vi "SS_Wait4Trigger.vi"(6 "Main Cluster IN":T1, 8 "Error In":errorcluster, 11 "Info In":string="\nWaiting for TimerScope Trigger\n- IN: SS TimerScope Trigger\n- OUT: SET SS ThermoRec Received Trigger\nPulse Number is 231123\nPulse Type is 4\n\nDuration (s) is  2.000000\nDelay (s)  is  1.000000\nScan Period (ms) is  15\nNumber of Samples is  134\n\nDelay Started\nDelay Complete\nExternal Measurement of Delay (s): 1.000000\nACQUIRING DATA") -> (0 "Error Out":errorcluster, 3 "Info Out":string="\nWaiting for TimerScope Trigger\n- IN: SS TimerScope Trigger\n- OUT: SET SS ThermoRec Received Trigger\nPulse Number is 231123\nPulse Type is 4\n\nDuration (s) is  2.000000\nDelay (s)  is  1.000000\nScan Period (ms) is  15\nNumber of Samples is  134\n\nDelay Started\nDelay Complete\nExternal Measurement of Delay (s): 1.000000\nACQUIRING DATA", 4 "Main Cluster OUT":T1)   [LabVIEW 2016]
uses:
  Control/Control_Main.ctl
  Control/Control_ModuleArray.ctl
  <vilib>/Platform/TimedLoop/XDataNode/timing_clust.ctl
  <vilib>/Platform/TimedLoop/XDataNode/nitl_modes.ctl
  <vilib>/Platform/TimedLoop/XDataNode/wakeup.ctl
  <vilib>/real-time/rtutility.llb/RT Restart Target (IP).vi
  <vilib>/Platform/TimedLoop/XDataNode/XDataNode.xnode
  <vilib>/Platform/TimedLoop/XDataNode/XDNodeRunTimeDep.lvlib
  <vilib>/real-time/NI_Real-Time Libraries.lvlib
panel:
  in  "Tab Control":enum32{"IN", "OUT", "SubVI Info"}(tab)
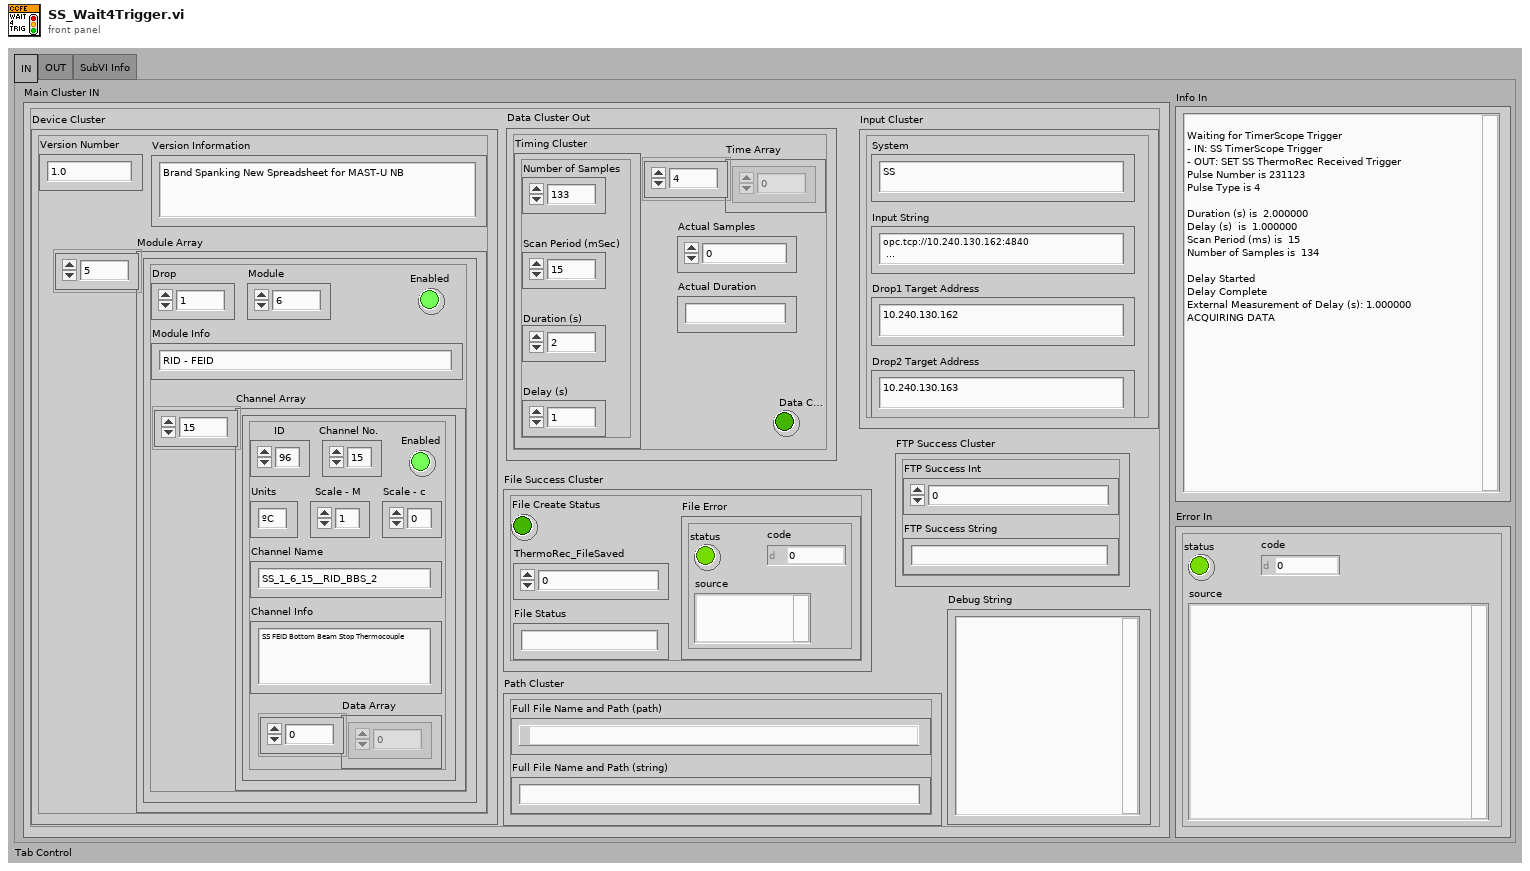
[diagram p1: front panel]
types:
  T1 = typedef "Control_Main.ctl" = cluster{"Device Cluster":cluster{"Module Array":T2, "Version Number":string, "Version Information":string}, "Input Cluster":cluster{"Input String":string, "Drop1 Target Address":string, "Drop2 Target Address":string, "System":string}, "Data Cluster Out":cluster{"Timing Cluster":cluster{"Number of Samples":i32, "Scan Period (mSec)":u32, "Duration (s)":dbl, "Delay (s)":dbl}, "Time Array":dbl[], "Actual Samples":i32, "Actual Duration":string, "Data Collection Error":bool}, "Path Cluster":cluster{"Full File Name and Path (path)":path, "Full File Name and Path (string)":string}, "File Success Cluster":cluster{"ThermoRec_FileSaved":i32, "File Create Status":bool, "File Error":errorcluster, "File Status":string}, "FTP Success Cluster":cluster{"FTP Success Int":i32, "FTP Success String":string}, "Debug String":string}
  T2 = typedef "Control_ModuleArray.ctl" = cluster{"Drop":i32, "Module":i32, "Module Info":string, "Enabled":bool, "Channel Array":cluster{"ID":i32, "Channel No.":i32, "Enabled":bool, "Channel Name":string, "Channel Info":string, "Units":string, "Scale - M":dbl, "Scale - c":dbl, "Data Array":dbl[]}[]}[]
  T3 = typedef "XDNodeRunTimeDep.lvlib/timing_clust.ctl" = cluster{"Expected End [f-1]":u64, "Actual End [f-1]":u64, "Finished Late? [f-1]":bool, "Expected End [i-1]":u64, "Actual End [i-1]":u64, "Finished Late? [i-1]":bool, "Expected Start [i]":u64, "Actual Start [i]":u64, "Expected Start [f]":u64, "Actual Start [f]":u64, "Source Name":string, "Structure Name":string, "Period":i64, "Deadline":i64, "Offset":i64, "Start":i64, "Priority":i32, "Timeout":i32, "Mode":T4, "Wakeup Reason":T5, "Error":errorcluster, "Source Type":string, "Secondary Source Type":string, "Global End Time":u64, "Global Start Time":u64, "Frame Duration":u64, "Iteration Duration":u64, "Assigned CPU":i32, "I/O Scan Engine Mode":u32}
  T4 = typedef "XDNodeRunTimeDep.lvlib/nitl_modes.ctl" = enum32{"No Change", "Process missed periods, maintain original phase", "Discard missed periods, maintain original phase", "Process missed periods, ignore original phase", "Discard missed periods, ignore original phase"}
  T5 = typedef "XDNodeRunTimeDep.lvlib/wakeup.ctl" = enum32{"Normal", "Aborted", "Asynchronous wakeup", "Timing source error", "Timed loop error", "Timeout"}
  T6 = cluster{"ID":i32, "Channel No.":i32, "Enabled":bool, "Channel Name":string, "Channel Info":string, "Units":string, "Scale - M":dbl, "Scale - c":dbl, "Data Array":dbl[]}[]
  T7 = cluster{"ID":i32, "Channel No.":i32, "Enabled":bool, "Channel Name":string, "Channel Info":string, "Units":string, "Scale - M":dbl, "Scale - c":dbl, "Data Array":dbl[]}
  T8 = cluster{"Drop":i32, "Module":i32, "Module Info":string, "Enabled":bool, "Channel Array":cluster{"ID":i32, "Channel No.":i32, "Enabled":bool, "Channel Name":string, "Channel Info":string, "Units":string, "Scale - M":dbl, "Scale - c":dbl, "Data Array":dbl[]}[]}
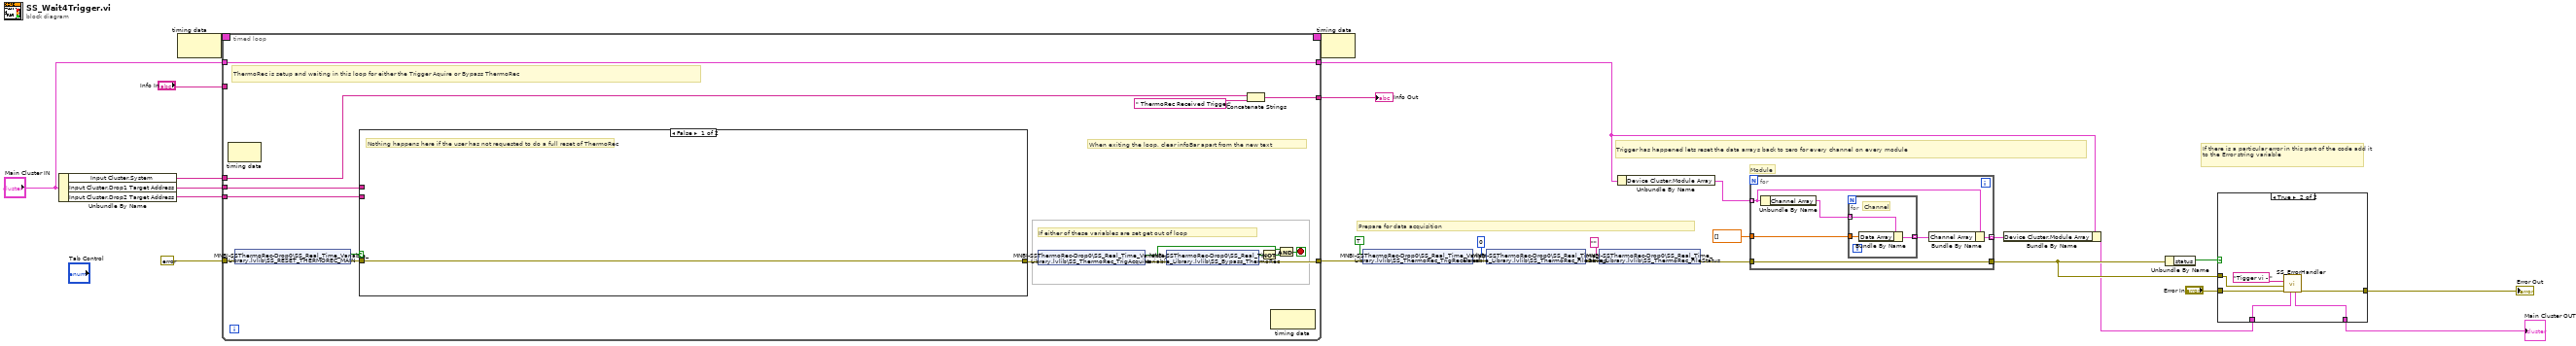
[diagram p0: block diagram]
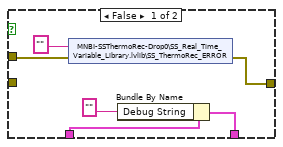
[diagram p2: hidden frame]
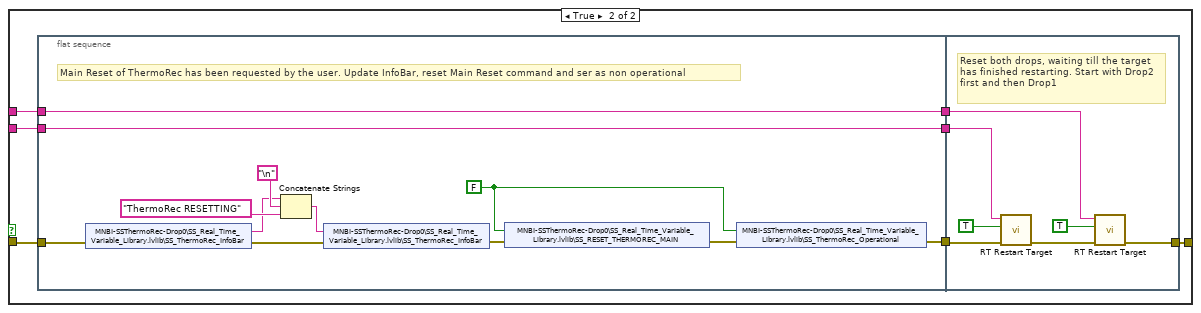
[diagram p3: hidden frame]
diagram:
  # "Trigger has happened lets reset the data arrays back to zero for every channel on every module"
  # "Module"
  # "Prepare for data acquisition"
  # "If there is a particular error in this part of the code add it to the Error string variable"
  n1 = Unbundle By Name("Main Cluster IN") -> ("Input Cluster.System"=w16:string, "Input Cluster.Drop1 Target Address"=w18:string, "Input Cluster.Drop2 Target Address"=w17:string)
  n2 = node-c288() -> (w26:T3)  [unwired: 1 in]
  n3 = timed-loop {
    timing: w26 -> [_]
    timing-out: [_] -> w25
    tunnel: [w36] -> w19
    tunnel: "Info In" -> [_]
    tunnel: [w42] -> w12
    tunnel: errorcluster {"status"=FALSE, "code"=0, "source"=""} ("error constant") -> [w34]
    tunnel: w18 -> [w31]
    tunnel: w17 -> [w30]
    tunnel: w16 -> [w28]
    tunnel: "Main Cluster IN" -> [w29]
    tunnel: [w29] -> w5
    stop <- w41 stop-if-true
    # "When exiting the loop, clear infoBar apart from the new text"
    # "If either of these variables are set get out of loop"
    # "ThermoRec is setup and waiting in this loop for either the Trigger Aquire or Bypass ThermoRec"
    n4 = node-c288() -> ()  [unwired: 1 in, 1 out]
    n5 = shared-variable "MNBI-SSThermoRec-Drop0\\SS_Real_Time_Variable_Library.lvlib\\SS_RESET_THERMOREC_MAIN"(error in=w34) -> (w39:bool, error out=w33:errorcluster)
    n6 = case shown="False" w39 {
      tunnel: w33 -> [w43 w49]
      tunnel: [w43 w48] -> w32
      tunnel: w31 -> [_ w46]
      tunnel: w30 -> [_ w44]
      frame False {
        # "Nothing happens here if the user has not requested to do a full reset of ThermoRec"
      }
      frame True {
        n7 = flat-sequence {
          tunnel: [w54] -> w50
          tunnel: w49 -> [w58]
          tunnel: [w53] -> w47
          tunnel: w46 -> [w53]
          tunnel: [w52] -> w45
          tunnel: w44 -> [w52]
          tunnel: w50 -> [w69]
          tunnel: [w64] -> w48
          tunnel: w47 -> [w63]
          tunnel: w45 -> [w68]
          frame #0 {
            w51 = FALSE ("SS_RESET_THERMOREC_MAIN")
            # "Main Reset of ThermoRec has been requested by the user. Update InfoBar, reset Main Reset command and ser as non operational"
            n8 = shared-variable "MNBI-SSThermoRec-Drop0\\SS_Real_Time_Variable_Library.lvlib\\SS_ThermoRec_InfoBar"(error in=w58) -> (w60:string, error out=w57:errorcluster)
            n9 = Concatenate Strings(w60, "\n", "ThermoRec RESETTING") -> (w59:string)
            n10 = shared-variable "MNBI-SSThermoRec-Drop0\\SS_Real_Time_Variable_Library.lvlib\\SS_ThermoRec_InfoBar"(w59, error in=w57) -> (error out=w56:errorcluster)
            n11 = shared-variable "MNBI-SSThermoRec-Drop0\\SS_Real_Time_Variable_Library.lvlib\\SS_RESET_THERMOREC_MAIN"(w51, error in=w56) -> (error out=w55:errorcluster)
            n12 = shared-variable "MNBI-SSThermoRec-Drop0\\SS_Real_Time_Variable_Library.lvlib\\SS_ThermoRec_Operational"(w51, error in=w55) -> (error out=w54:errorcluster)
          }
          frame #1 {
            # "Reset both drops, waiting till the target has finished restarting. Start with Drop2 first and then Drop1"
            n13 = call-poly <vilib>:"RT Restart Target.vi"("error in (no error)"=w69, "wait for restart? (F)"=TRUE, "target address"=w68) -> ("error out"=w65:errorcluster)  [unwired: 6 in, 2 out]
            n14 = call-poly <vilib>:"RT Restart Target.vi"("error in (no error)"=w65, "wait for restart? (F)"=TRUE, "target address"=w63) -> ("error out"=w64:errorcluster)  [unwired: 6 in, 2 out]
          }
        }
      }
    }
    n15 = shared-variable "MNBI-SSThermoRec-Drop0\\SS_Real_Time_Variable_Library.lvlib\\SS_ThermoRec_TrigAcquire"(error in=w32) -> (w38:bool, error out=w35:errorcluster)
    n16 = shared-variable "MNBI-SSThermoRec-Drop0\\SS_Real_Time_Variable_Library.lvlib\\SS_Bypass_ThermoRec"(error in=w35) -> (w37:bool, error out=w36:errorcluster)
    n17 = Concatenate Strings(w28, " ThermoRec Received Trigger") -> (w42:string)
    n18 = Not(x=w37) -> (.not. x?=w40:bool)
    n19 = node-c288() -> ()  [unwired: 1 in, 1 out]
    n20 = And(x=w38, y=w40) -> (x .and. y?=w41:bool)
  }
  "Info Out" <- w12
  n21 = node-c288(w25) -> ()  [unwired: 1 out]
  n22 = shared-variable "MNBI-SSThermoRec-Drop0\\SS_Real_Time_Variable_Library.lvlib\\SS_ThermoRec_TrigReceived"(TRUE, error in=w19) -> (error out=w24:errorcluster)
  n23 = shared-variable "MNBI-SSThermoRec-Drop0\\SS_Real_Time_Variable_Library.lvlib\\SS_ThermoRec_FileSaved"(0 ("SS_ThermoRec_FileSaved"), error in=w24) -> (error out=w23:errorcluster)
  n24 = shared-variable "MNBI-SSThermoRec-Drop0\\SS_Real_Time_Variable_Library.lvlib\\SS_ThermoRec_FileStatus"("" ("SS_ThermoRec_FileStatus"), error in=w23) -> (error out=w4:errorcluster)
  n25 = Unbundle By Name(w5) -> ("Device Cluster.Module Array"=w9:T2)
  n26 = for {
    tunnel: w9 -> [w74] mode=indexing
    tunnel: dbl[] [] -> [w76]
    tunnel: [w73] -> w7 mode=indexing
    tunnel: w4 -> [w72]
    tunnel: [w72] -> w3
    n27 = Unbundle By Name(w74) -> ("Channel Array"=w77:T6)
    n28 = for {
      tunnel: w77 -> [w79] mode=indexing
      tunnel: w76 -> [w80]
      tunnel: [w78] -> w75 mode=indexing
      # "Channel"
      n29 = Bundle By Name(cluster=w79, "Data Array"=w80) -> (w78:T7)
    }
    n30 = Bundle By Name(cluster=w74, "Channel Array"=w75) -> (w73:T8)
  }
  n31 = Bundle By Name(cluster=w5, "Device Cluster.Module Array"=w7) -> (w2:T1)
  n32 = Unbundle By Name(w3) -> ("status"=w14:bool)
  n33 = case shown="True" w14 {
    tunnel: w3 -> [w86 w87]
    tunnel: [w84 w92] -> w11
    tunnel: "Error In" -> [_ w91]
    tunnel: w2 -> [w83 w89]
    tunnel: [w82 w88] -> w1
    frame False {
      n34 = shared-variable "MNBI-SSThermoRec-Drop0\\SS_Real_Time_Variable_Library.lvlib\\SS_ThermoRec_ERROR"("", error in=w86) -> (error out=w84:errorcluster)
      n35 = Bundle By Name(cluster=w83, "Debug String"="") -> (w82:T1)
    }
    frame True {
      n36 = call "SS_ErrorHandler.vi"("Main Cluster IN"=w89, "Error In"=w91, "SubVI Error"=w87, "SubVI Name"="Tigger vi - ") -> ("Error Out"=w92:errorcluster, "Main Cluster OUT"=w88:T1)  [unwired: 5 in, 1 out]
    }
  }
  "Error Out" <- w11
  "Main Cluster OUT" <- w1
